vi "two_joysticks_without_sensors.vi"() -> ()   [LabVIEW 2019]
uses:
  <vilib>/addons/eal4LabVIEW/ApiLib/Connection control/ealApiConnect_string.vi
  <vilib>/Utility/inputDevices.llb/joystickAcquire.vi
  <vilib>/Utility/inputDevices.llb/closeJoystick.vi
  <vilib>/addons/eal4LabVIEW/eal4LabVIEW.lvlib
panel:
  out "x-y":u32
  out "error out":errorcluster
  out "axis info 2":T1
  out "Numeric 2":dbl
  out "axis info":T1
  out "Numeric 3":dbl
  out "Boom":dbl(slide) scale=-500.0..500.0
  in  "parameters set 3":T2
  out "Arm":dbl(slide) scale=-500.0..500.0
  in  "parameters set 2":T2
  out "Numeric":dbl
  out "Bucket":dbl(slide) scale=-500.0..500.0
  in  "parameters set":T2
  in  "condition 3":i32(ring) items=["AXIS_CONDITION_ACTIVE"=0, "AXIS_CONDITION_PARKING"=1, "AXIS_CONDITION_DEACTIVATED"=2, "AXIS_CONDITION_ACTIVE_DECOUPLED"=4, "AXIS_CONDITION_PARKING_DECOUPLED"=5, "AXIS_CONDITION_DEACTIVATED_DECOUPLED"=6, "AXIS_CONDITION_ACTIVE_PARAMETERIZATION"=8, "AXIS_CONDITION_PARKING_PARAMETERIZATION"=9, "AXIS_CONDITION_DEACTIVATED_PARAMETERIZATION"=10, "AXIS_CONDITION_ACTIVE_DECOUPLED_PARAMETERIZATION"=12, "AXIS_CONDITION_PARKING_DECOUPLED_PARAMETERIZATION"=13, "AXIS_CONDITION_DEACTIVATED_DECOUPLED_PARAMETERIZATION"=14]
  in  "slave index 3":i32
  in  "condition 2":i32(ring) items=["AXIS_CONDITION_ACTIVE"=0, "AXIS_CONDITION_PARKING"=1, "AXIS_CONDITION_DEACTIVATED"=2, "AXIS_CONDITION_ACTIVE_DECOUPLED"=4, "AXIS_CONDITION_PARKING_DECOUPLED"=5, "AXIS_CONDITION_DEACTIVATED_DECOUPLED"=6, "AXIS_CONDITION_ACTIVE_PARAMETERIZATION"=8, "AXIS_CONDITION_PARKING_PARAMETERIZATION"=9, "AXIS_CONDITION_DEACTIVATED_PARAMETERIZATION"=10, "AXIS_CONDITION_ACTIVE_DECOUPLED_PARAMETERIZATION"=12, "AXIS_CONDITION_PARKING_DECOUPLED_PARAMETERIZATION"=13, "AXIS_CONDITION_DEACTIVATED_DECOUPLED_PARAMETERIZATION"=14]
  in  "slave index 2":i32
  in  "condition":i32(ring) items=["AXIS_CONDITION_ACTIVE"=0, "AXIS_CONDITION_PARKING"=1, "AXIS_CONDITION_DEACTIVATED"=2, "AXIS_CONDITION_ACTIVE_DECOUPLED"=4, "AXIS_CONDITION_PARKING_DECOUPLED"=5, "AXIS_CONDITION_DEACTIVATED_DECOUPLED"=6, "AXIS_CONDITION_ACTIVE_PARAMETERIZATION"=8, "AXIS_CONDITION_PARKING_PARAMETERIZATION"=9, "AXIS_CONDITION_DEACTIVATED_PARAMETERIZATION"=10, "AXIS_CONDITION_ACTIVE_DECOUPLED_PARAMETERIZATION"=12, "AXIS_CONDITION_PARKING_DECOUPLED_PARAMETERIZATION"=13, "AXIS_CONDITION_DEACTIVATED_DECOUPLED_PARAMETERIZATION"=14]
  in  "slave index":i32
  in  "stop":bool
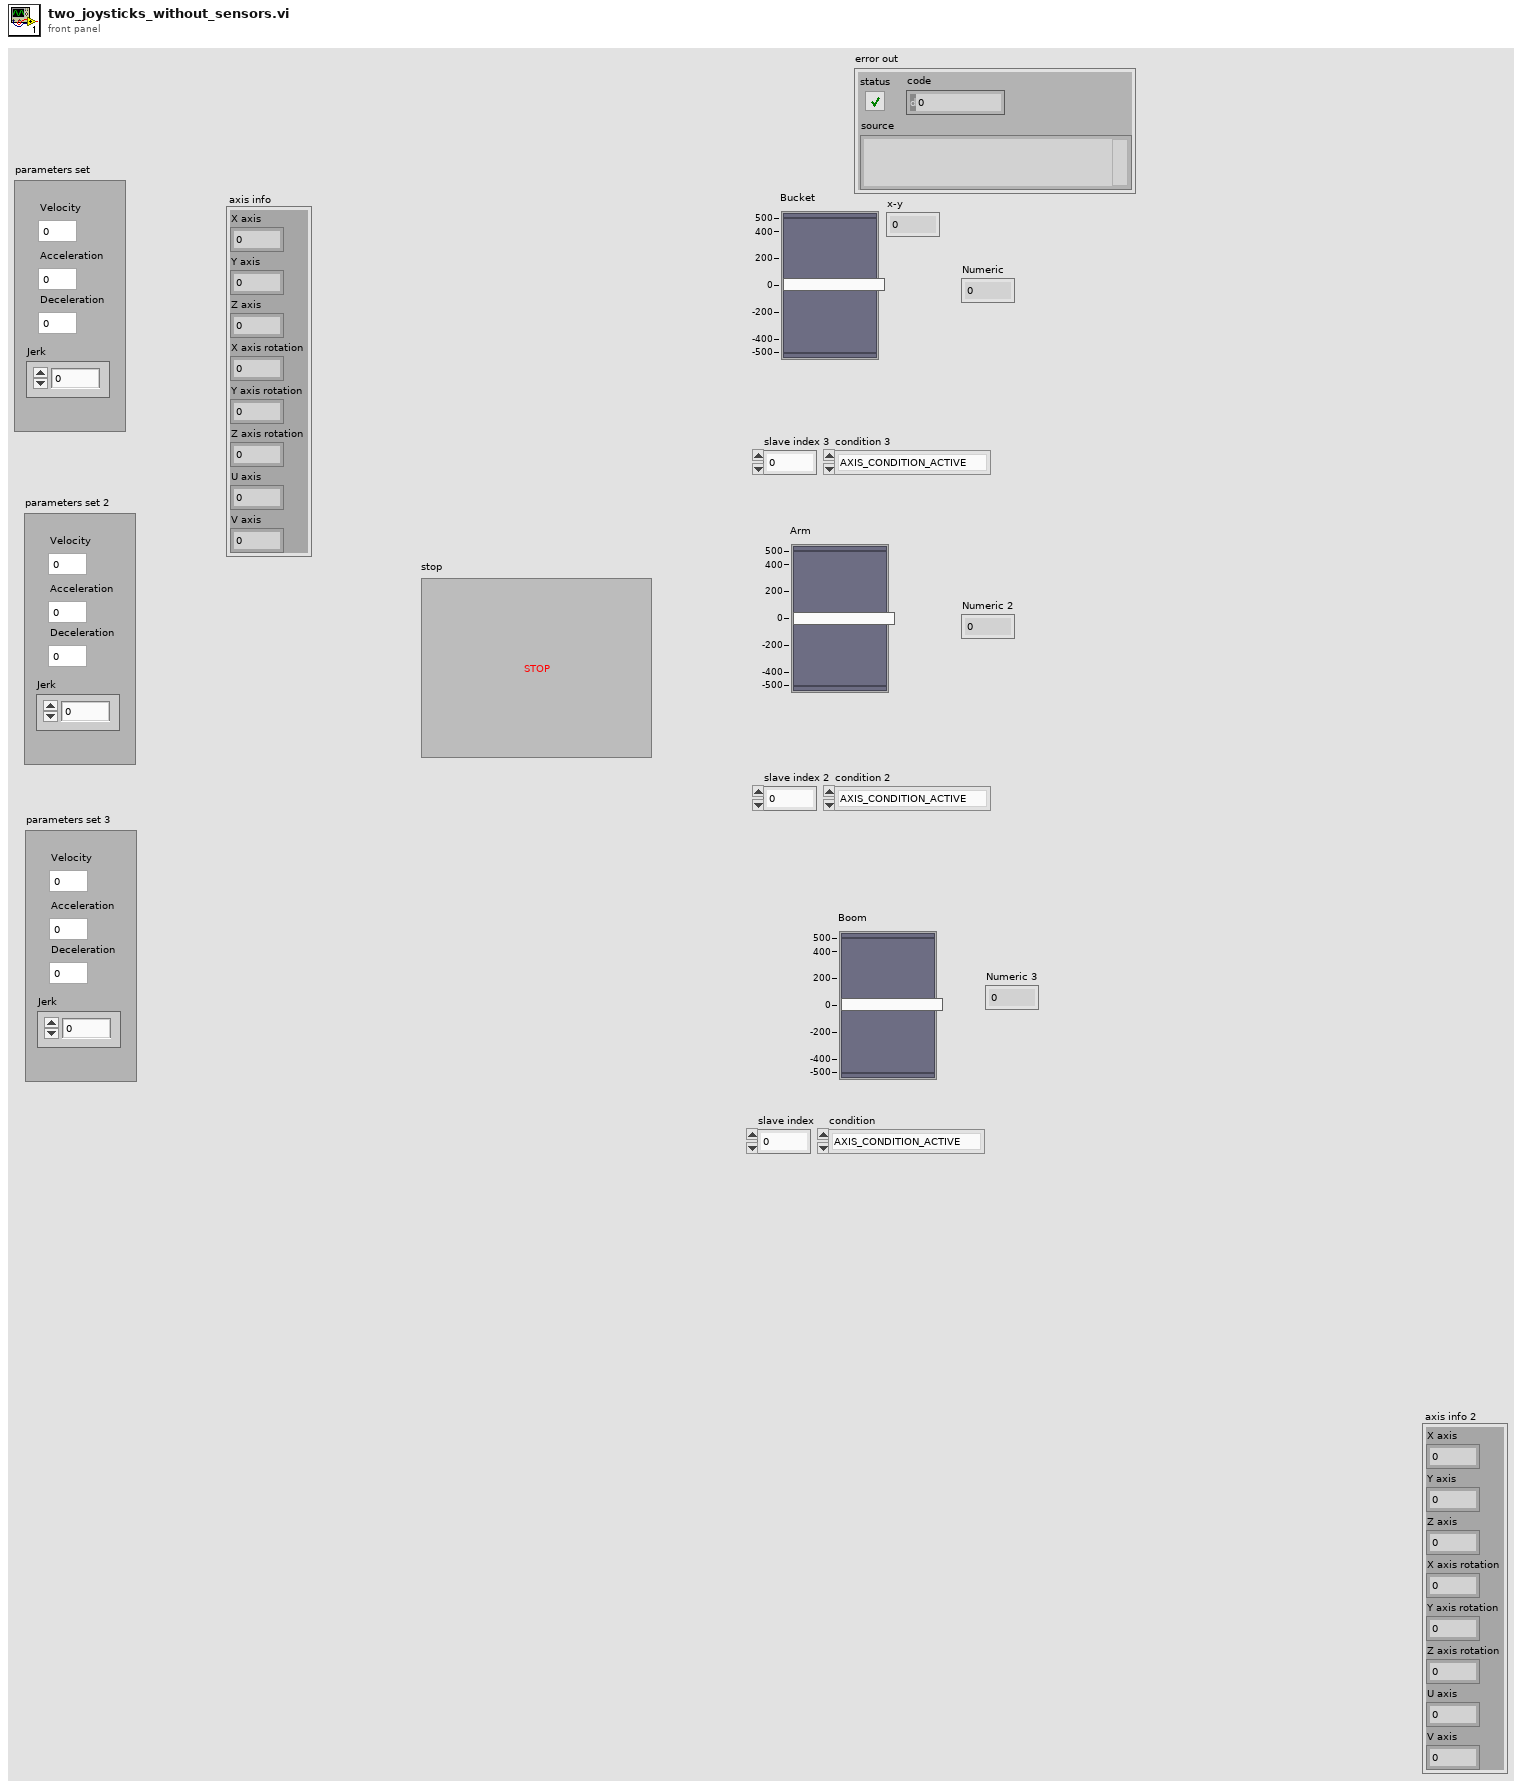
[diagram p1: front panel]
types:
  T1 = cluster{"X axis":i32, "Y axis":i32, "Z axis":i32, "X axis rotation":i32, "Y axis rotation":i32, "Z axis rotation":i32, "U axis":i32, "V axis":i32}
  T2 = cluster{"Velocity":dbl, "Acceleration":dbl, "Deceleration":dbl, "Jerk":dbl}
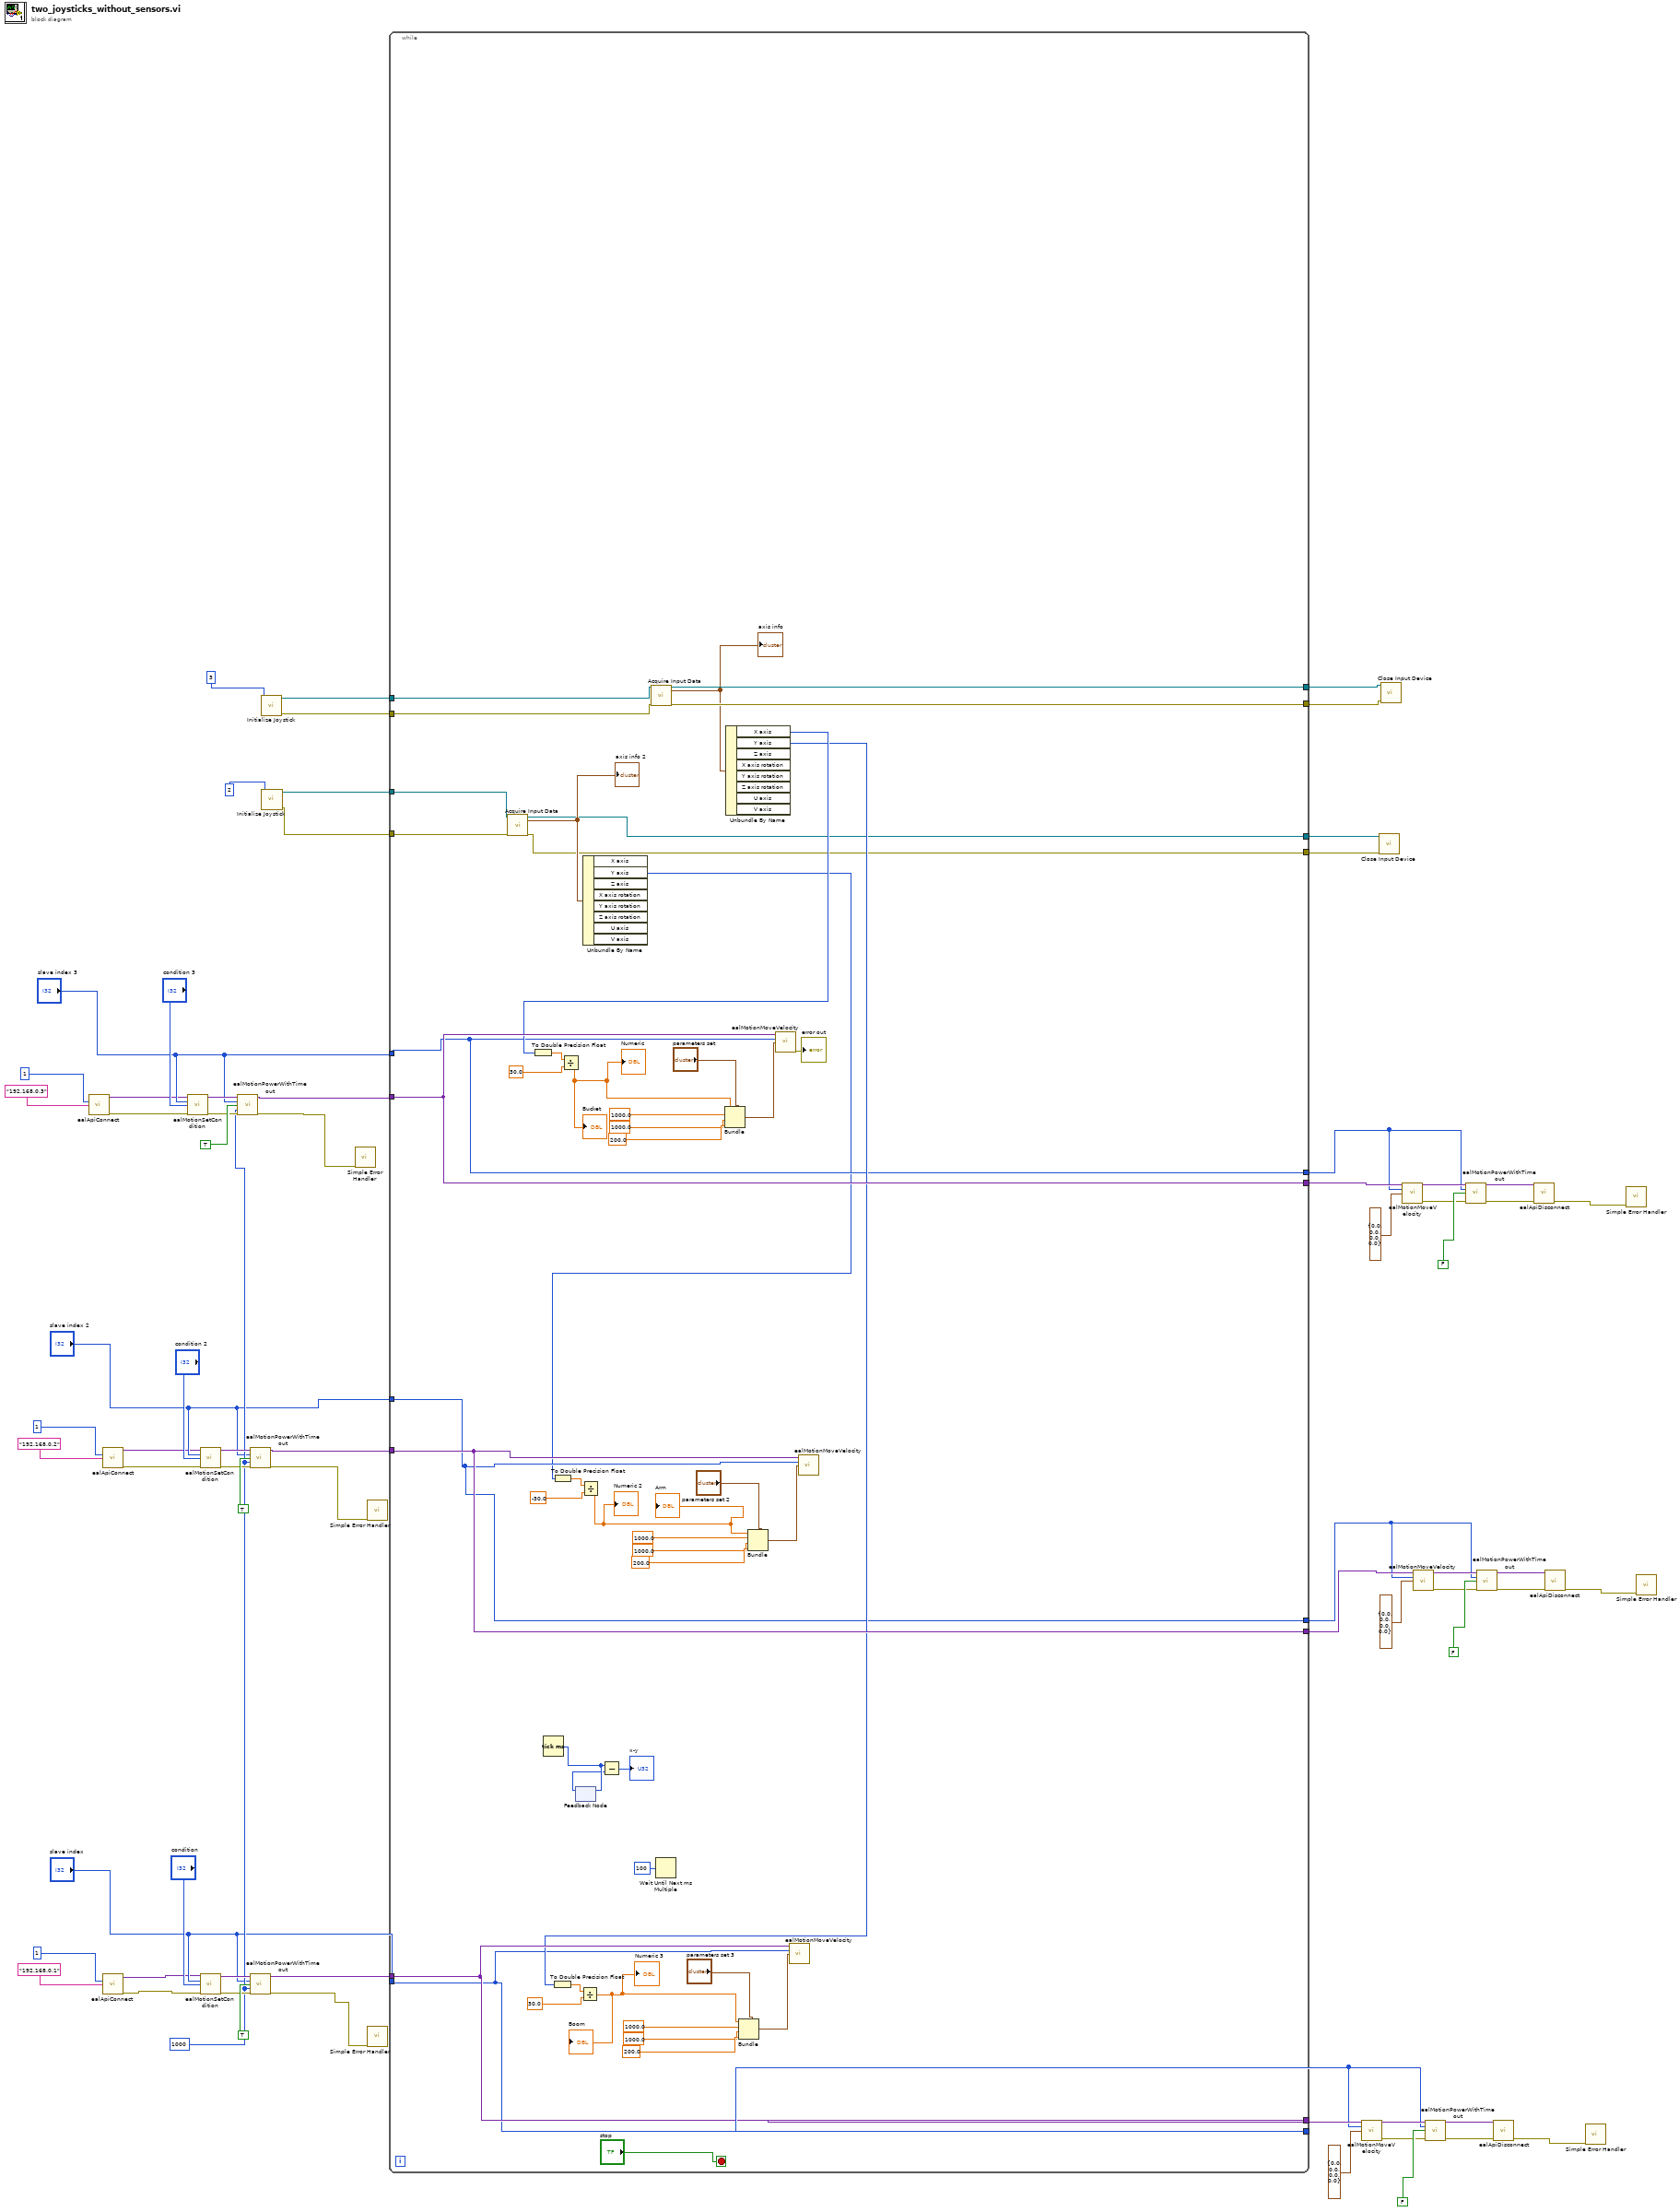
[diagram p0: block diagram]
diagram:
  w26 = 1000
  n1 = call-poly <vilib>:"ealApiConnect.vi"("maximum no of axes"=1, "ip address"="192.168.0.3") -> ("connection out"=w11:variant, "error out"=w12:errorcluster)  [unwired: 12 in]
  n2 = call-poly <vilib>:"ealApiConnect.vi"("maximum no of axes"=1, "ip address"="192.168.0.1") -> ("connection out"=w16:variant, "error out"=w15:errorcluster)  [unwired: 12 in]
  n3 = call-poly <vilib>:"ealApiConnect.vi"("maximum no of axes"=1, "ip address"="192.168.0.2") -> ("connection out"=w14:variant, "error out"=w13:errorcluster)  [unwired: 12 in]
  n4 = call <vilib>:"ealMotionSetCondition.vi"("connection in"=w11, "slave index"="slave index 3", "condition"="condition 3", "error in (no error)"=w12) -> ("connection out"=w46:variant, "error out"=w47:errorcluster)  [unwired: 10 in]
  n5 = call <vilib>:"ealMotionSetCondition.vi"("connection in"=w14, "slave index"="slave index 2", "condition"="condition 2", "error in (no error)"=w13) -> ("connection out"=w52:variant, "error out"=w53:errorcluster)  [unwired: 10 in]
  n6 = call <vilib>:"ealMotionSetCondition.vi"("connection in"=w16, "slave index"="slave index", "condition"="condition", "error in (no error)"=w15) -> ("connection out"=w57:variant, "error out"=w58:errorcluster)  [unwired: 10 in]
  n7 = call <vilib>:"ealMotionPowerWithTimeout.vi"("connection in"=w46, "slave index"="slave index 3", "value"=TRUE, "timeout"=w26, "error in (no error)"=w47) -> ("connection out"=w21:variant, "error out"=w20:errorcluster)  [unwired: 9 in]
  n8 = call <vilib>:"ealMotionPowerWithTimeout.vi"("connection in"=w52, "slave index"="slave index 2", "value"=TRUE, "timeout"=w26, "error in (no error)"=w53) -> ("connection out"=w23:variant, "error out"=w22:errorcluster)  [unwired: 9 in]
  n9 = call <vilib>:"ealMotionPowerWithTimeout.vi"("connection in"=w57, "slave index"="slave index", "value"=TRUE, "timeout"=w26, "error in (no error)"=w58) -> ("connection out"=w25:variant, "error out"=w24:errorcluster)  [unwired: 9 in]
  n10 = call <vilib>:"Initialize Joystick.vi"("device index"=3) -> ("error out"=w8:errorcluster, "device ID"=w9:refnum<k1>)  [unwired: 9 in]
  n11 = call <vilib>:"Initialize Joystick.vi"("device index"=2 ("device index 2")) -> ("error out"=w3:errorcluster, "device ID"=w4:refnum<k1>)  [unwired: 9 in]
  n12 = call <vilib>:"Simple Error Handler.vi"("error in (no error)"=w20) -> ()  [unwired: 4 in, 5 out]
  n13 = call <vilib>:"Simple Error Handler.vi"("error in (no error)"=w22) -> ()  [unwired: 4 in, 5 out]
  n14 = call <vilib>:"Simple Error Handler.vi"("error in (no error)"=w24) -> ()  [unwired: 4 in, 5 out]
  n15 = while {
    tunnel: w25 -> [w102]
    tunnel: "slave index" -> [w86]
    tunnel: [w102] -> w69
    tunnel: [w86] -> w60
    tunnel: w23 -> [w108]
    tunnel: "slave index 2" -> [w88]
    tunnel: w21 -> [w119]
    tunnel: "slave index 3" -> [w87]
    tunnel: [w119] -> w31
    tunnel: [w87] -> w30
    tunnel: [w108] -> w29
    tunnel: [w88] -> w28
    tunnel: w9 -> [w101]
    tunnel: w8 -> [w100]
    tunnel: [w99] -> w7
    tunnel: [w98] -> w6
    tunnel: w4 -> [w81]
    tunnel: w3 -> [w80]
    tunnel: [w79] -> w2
    tunnel: [w78] -> w1
    stop <- "stop" stop-if-true
    n16 = call-poly <vilib>:"Acquire Input Data.vi"("device ID"=w81, "error in (no error)"=w80) -> ("device ID"=w79:refnum<k1>, "axis info"=w82:T1, "error out"=w78:errorcluster)  [unwired: 13 in, 2 out]
    "axis info 2" <- w82
    n17 = Tick Count (ms)() -> (millisecond timer value=w75:u32)
    n18 = feedback-in #1(w75) -> ()
    n19 = feedback #1() -> (w74:u32)  [unwired: 1 in]
    n20 = Unbundle By Name(w82) -> ("Y axis"=w77:i32)  [unwired: 7 out]
    n21 = To Double Precision Float(number=w77) -> (double precision float=w84:dbl)
    n22 = Divide(x=w84, y=-30.0) -> (x/y=w83:dbl)
    "Arm" <- w83
    "Numeric 2" <- w83
    n23 = Subtract(x=w75, y=w74) -> (x-y=→"x-y":u32)
    n24 = call-poly <vilib>:"Acquire Input Data.vi"("device ID"=w101, "error in (no error)"=w100) -> ("device ID"=w98:refnum<k1>, "axis info"=w97:T1, "error out"=w99:errorcluster)  [unwired: 13 in, 2 out]
    "axis info" <- w97
    n25 = Wait Until Next ms Multiple(millisecond multiple=u32 100) -> ()  [unwired: 1 out]
    n26 = Unbundle By Name(w97) -> ("X axis"=w94:i32, "Y axis"=w90:i32)  [unwired: 6 out]
    n27 = To Double Precision Float(number=w94) -> (double precision float=w95:dbl)
    n28 = To Double Precision Float(number=w90) -> (double precision float=w91:dbl)
    n29 = Divide(x=w95, y=30.0) -> (x/y=w93:dbl)
    "Bucket" <- w93
    "Numeric" <- w93
    n30 = Divide(x=w91, y=30.0) -> (x/y=w89:dbl)
    "Boom" <- w89
    "Numeric 3" <- w89
    n31 = Bundle(cluster="parameters set", "Velocity"=w93, "Acceleration"=1000.0, "Deceleration"=1000.0, "Jerk"=200.0) -> (w116:T2)
    n32 = Bundle(cluster="parameters set 3", "Velocity"=w89, "Acceleration"=1000.0, "Deceleration"=1000.0, "Jerk"=200.0) -> (w105:T2)
    n33 = Bundle(cluster="parameters set 2", "Velocity"=w83, "Acceleration"=1000.0, "Deceleration"=1000.0, "Jerk"=200.0) -> (w111:T2)
    n34 = call <vilib>:"ealMotionMoveVelocity.vi"("connection in"=w119, "slave index"=w87, "parameters set"=w116) -> ("error out"=→"error out":errorcluster)  [unwired: 11 in, 1 out]
    n35 = call <vilib>:"ealMotionMoveVelocity.vi"("connection in"=w102, "slave index"=w86, "parameters set"=w105) -> ()  [unwired: 11 in, 2 out]
    n36 = call <vilib>:"ealMotionMoveVelocity.vi"("connection in"=w108, "slave index"=w88, "parameters set"=w111) -> ()  [unwired: 11 in, 2 out]
  }
  n37 = call <vilib>:"ealMotionMoveVelocity.vi"("connection in"=w69, "slave index"=w60, "parameters set"=T2 {"Velocity"=0.0, "Acceleration"=0.0, "Deceleration"=0.0, "Jerk"=0.0}) -> ("connection out"=w65:variant, "error out"=w62:errorcluster)  [unwired: 11 in]
  n38 = call-poly <vilib>:"Close Input Device.vi"("error in (no error)"=w1, "device ID"=w2) -> ()  [unwired: 8 in, 1 out]
  n39 = call-poly <vilib>:"Close Input Device.vi"("error in (no error)"=w7, "device ID"=w6) -> ()  [unwired: 8 in, 1 out]
  n40 = call <vilib>:"ealMotionMoveVelocity.vi"("connection in"=w31, "slave index"=w30, "parameters set"=T2 {"Velocity"=0.0, "Acceleration"=0.0, "Deceleration"=0.0, "Jerk"=0.0}) -> ("connection out"=w36:variant, "error out"=w33:errorcluster)  [unwired: 11 in]
  n41 = call <vilib>:"ealMotionMoveVelocity.vi"("connection in"=w29, "slave index"=w28, "parameters set"=T2 {"Velocity"=0.0, "Acceleration"=0.0, "Deceleration"=0.0, "Jerk"=0.0}) -> ("connection out"=w43:variant, "error out"=w40:errorcluster)  [unwired: 11 in]
  n42 = call <vilib>:"ealMotionPowerWithTimeout.vi"("connection in"=w65, "slave index"=w60, "value"=FALSE, "error in (no error)"=w62) -> ("connection out"=w64:variant, "error out"=w63:errorcluster)  [unwired: 10 in]
  n43 = call <vilib>:"ealMotionPowerWithTimeout.vi"("connection in"=w36, "slave index"=w30, "value"=FALSE, "error in (no error)"=w33) -> ("connection out"=w35:variant, "error out"=w34:errorcluster)  [unwired: 10 in]
  n44 = call <vilib>:"ealMotionPowerWithTimeout.vi"("connection in"=w43, "slave index"=w28, "value"=FALSE, "error in (no error)"=w40) -> ("connection out"=w42:variant, "error out"=w41:errorcluster)  [unwired: 10 in]
  n45 = call <vilib>:"ealApiDisconnect.vi"("connection in"=w64, "error in (no error)"=w63) -> ("error out"=w61:errorcluster)  [unwired: 13 in]
  n46 = call <vilib>:"ealApiDisconnect.vi"("connection in"=w35, "error in (no error)"=w34) -> ("error out"=w32:errorcluster)  [unwired: 13 in]
  n47 = call <vilib>:"ealApiDisconnect.vi"("connection in"=w42, "error in (no error)"=w41) -> ("error out"=w39:errorcluster)  [unwired: 13 in]
  n48 = call <vilib>:"Simple Error Handler.vi"("error in (no error)"=w61) -> ()  [unwired: 4 in, 5 out]
  n49 = call <vilib>:"Simple Error Handler.vi"("error in (no error)"=w32) -> ()  [unwired: 4 in, 5 out]
  n50 = call <vilib>:"Simple Error Handler.vi"("error in (no error)"=w39) -> ()  [unwired: 4 in, 5 out]
